vi "initialization.vi"(8 "error in (no error)":errorcluster, 11 "DLOwis in":refnum<class "DLOwis.lvclass">) -> (0 "error out":errorcluster, 3 "DLOwis out":refnum<class "DLOwis.lvclass">)   [LabVIEW 2020, in "DLOwis.lvclass"]
uses:
  DLOwis.lvclass
  C:/dev/TRANCON/Classes/GeneralFunctionality/GeneralFunctionality.lvclass
  C:/dev/TRANCON/Classes/Delay Line/DelayLine.lvclass
  GeneralFunctionality/GeneralFunctionality.lvclass/GeneralFunctionality.ctl
  DelayLine.lvclass/DelayLine.ctl
  dependecies/globalVarII.vi
  <vilib>/Utility/libraryn.llb/Check if File or Folder Exists.vi
  <vilib>/Utility/error.llb/Error Cluster From Error Code.vi
  Config/Config.lvclass
  DelayLine.lvclass
  GeneralFunctionality/GeneralFunctionality.lvclass
panel:
  in  "Init file":string="config_ligne_à_retard.ls"
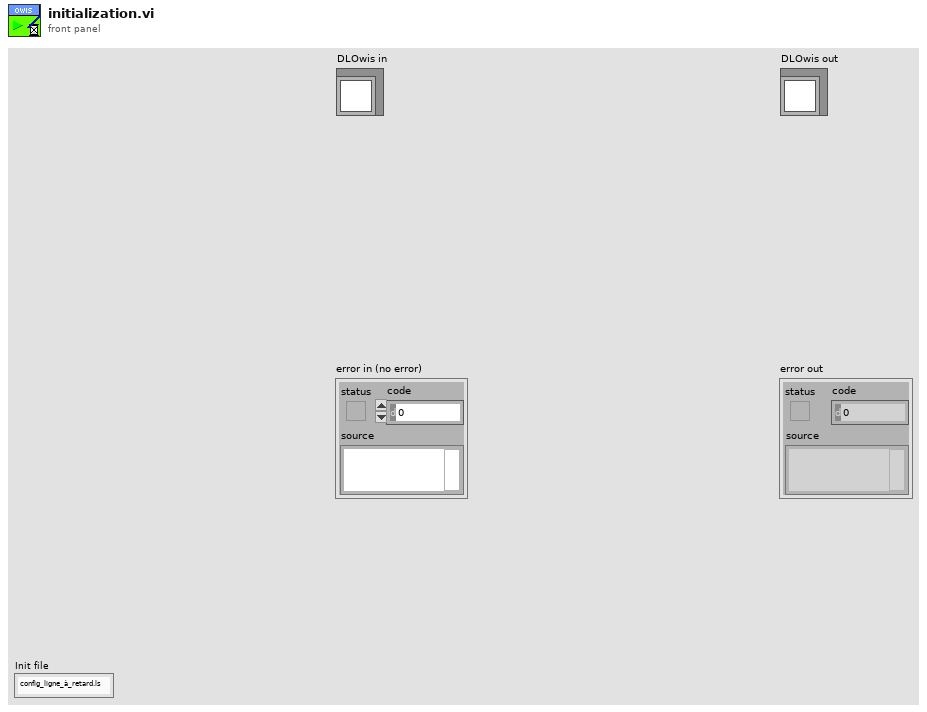
[diagram p1: front panel]
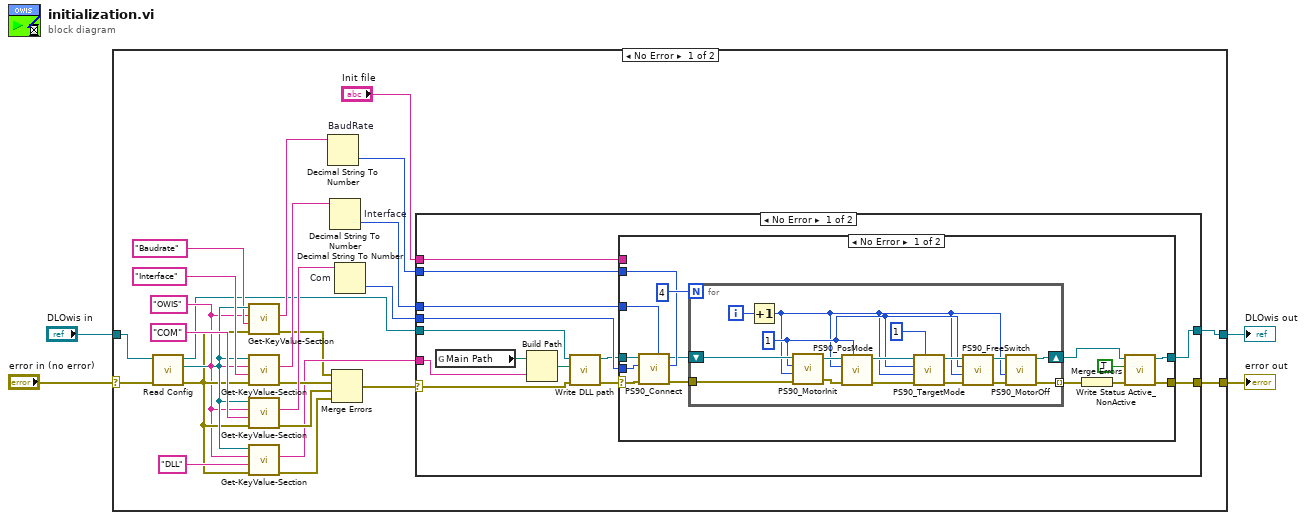
[diagram p0: block diagram]
diagram:
  n1 = case shown="No Error" "error in (no error)" {
    selector: "error in (no error)" -> [w6 w78]
    tunnel: "DLOwis in" -> [w29 w77]
    tunnel: [w7 w78] -> w4
    tunnel: [w5 w77] -> w3
    frame No Error {
      w11 = "OWIS" ("Section")
      n2 = call "Read Config.vi"("error in (no error)"=w6, "GeneralFunctionality en entrée"=w29) -> ("error out"=w14:errorcluster, "Config.lvclass"=w15:refnum<class "Config.lvclass">, "GeneralFunctionality en sortie"=w8:refnum<class "DLOwis.lvclass">)  [unwired: 7 in]
      n3 = call-dynamic "Get-KeyValue-Section.vi"("error in (no error)"=w14, "Key"="Baudrate" ("y"), "Section"=w11, "Config in"=w15) -> ("error out"=w13:errorcluster, "Value"=w10:string)  [unwired: 5 in, 1 out]
      n4 = call-dynamic "Get-KeyValue-Section.vi"("error in (no error)"=w14, "Key"="Interface", "Section"=w11, "Config in"=w15) -> ("error out"=w23:errorcluster, "Value"=w20:string)  [unwired: 5 in, 1 out]
      n5 = call-dynamic "Get-KeyValue-Section.vi"("error in (no error)"=w14, "Key"="COM", "Section"=w11, "Config in"=w15) -> ("error out"=w22:errorcluster, "Value"=w25:string)  [unwired: 5 in, 1 out]
      n6 = call-dynamic "Get-KeyValue-Section.vi"("error in (no error)"=w14, "Key"="DLL", "Section"=w11, "Config in"=w15) -> ("error out"=w18:errorcluster, "Value"=w16:string)  [unwired: 5 in, 1 out]
      n7 = Decimal String To Number "BaudRate"(string=w10) -> (number=w9:i32)  [unwired: 2 in, 1 out]
      n8 = Decimal String To Number "Interface"(string=w20) -> (number=w19:i32)  [unwired: 2 in, 1 out]
      n9 = Merge Errors(w13, w23, w22, w18) -> (w21:errorcluster)
      n10 = Decimal String To Number "Com"(string=w25) -> (number=w24:i32)  [unwired: 2 in, 1 out]
      n11 = case shown="No Error" w21 {
        selector: w21 -> [w30 w76]
        tunnel: [w38 w76] -> w7
        tunnel: [w39 w75] -> w5
        tunnel: w8 -> [w32 w75]
        tunnel: "Init file" -> [w42 _]
        tunnel: w19 -> [w41 _]
        tunnel: w24 -> [w40 _]
        tunnel: w16 -> [w34 _]
        tunnel: w9 -> [w33 _]
        frame No Error {
          n12 = global read "globalVarII.vi" "Main Path"() -> (w37:path)
          n13 = Build Path(base path=w37, name or relative path=w34) -> (appended path=w31:path)
          n14 = call "Write DLL path.vi"("error in (no error)"=w30, "DLL path"=w31, "DelayLine in"=w32) -> ("error out"=w35:errorcluster, "DelayLine out"=w36:refnum<class "DLOwis.lvclass">)  [unwired: 7 in]
          n15 = case shown="No Error" w35 {
            selector: w35 -> [w51 w73]
            tunnel: w42 -> [_ _]
            tunnel: w41 -> [w45 _]
            tunnel: w40 -> [w46 _]
            tunnel: [w56 w74] -> w39
            tunnel: [w55 w73] -> w38
            tunnel: w36 -> [w52 w74]
            tunnel: w33 -> [w47 _]
            frame No Error {
              n16 = call "PS90_Connect.vi"("par2"=w47, "Interface"=w45, "error in (no error)"=w51, "par1"=w46, "DLOwis.lvclass"=w52) -> ("error out"=w44:errorcluster, "DLOwis.lvclass"=w43:refnum<class "DLOwis.lvclass">)  [unwired: 5 in]
              n17 = for {
                N: 4 -> [_]
                shift-right: [w60] -> w50
                shift-left: w43 -> [w67]
                tunnel: w44 -> [w66]
                tunnel: [w59] -> w49 mode=indexing
                i -> [w58]
                w65 = 1 ("Control unit ID")
                n18 = Increment(x=w58) -> (x+1=w57:i32)
                n19 = call "PS90_MotorInit.vi"("error in (no error)"=w66, "Axis number"=w57, "Control unit ID"=w65, "DLOwis.lvclass"=w67) -> ("error out"=w63:errorcluster, "DLOwis.lvclass"=w64:refnum<class "DLOwis.lvclass">)  [unwired: 1 in]
                n20 = call "PS90_PosMode.vi"("Control unit ID"=w65, "error in (no error)"=w63, "Axis number"=w57, "DLOwis.lvclass"=w64) -> ("error out"=w70:errorcluster, "DLOwis.lvclass"=w71:refnum<class "DLOwis.lvclass">)  [unwired: 5 in, 1 out]
                n21 = call "PS90_TargetMode.vi"("Value-In"=1, "error in (no error)"=w70, "Axis number"=w57, "Control unit ID"=w65, "DLOwis.lvclass"=w71) -> ("error out"=w69:errorcluster, "DLOwis.lvclass"=w72:refnum<class "DLOwis.lvclass">)  [unwired: 2 in, 1 out]
                n22 = call "PS90_FreeSwitch.vi"("error in (no error)"=w69, "Axis number"=w57, "Control unit ID"=w65, "DLOwis.lvclass"=w72) -> ("error out"=w62:errorcluster, "DLOwis.lvclass"=w61:refnum<class "DLOwis.lvclass">)  [unwired: 6 in]
                n23 = call "PS90_MotorOff.vi"("error in (no error)"=w62, "Axis number"=w57, "DLOwis.lvclass"=w61) -> ("error out"=w59:errorcluster, "DLOwis.lvclass"=w60:refnum<class "DLOwis.lvclass">)  [unwired: 7 in]
              }
              n24 = Merge Errors(w49) -> (w48:errorcluster)
              n25 = call "Write Status Active_NonActive.vi"("error in (no error)"=w48, "Status Active/NonActive"=TRUE, "GeneralFunctionality in"=w50) -> ("error out"=w55:errorcluster, "GeneralFunctionality out"=w56:refnum<class "DLOwis.lvclass">)  [unwired: 7 in]
            }
            frame Error {
            }
          }
        }
        frame Error {
        }
      }
    }
    frame Error {
    }
  }
  "error out" <- w4
  "DLOwis out" <- w3
